vi "LabelNodeConfig.vi"(4 "State In":T1={"Name"="...", "Hash"=0, "Type"=enum."I32"}) -> (0 "Canceled?":bool, 1 "State Out":T1={"Name"="...", "Hash"=0, "Type"=enum."I32"})   [LabVIEW 2012]
uses:
  ScriptingSupport/PictureRing.ctl
  State.ctl
  Core/Master Types.ctl
  CRef.lvlib
  CRef Label Node.xnode
panel:
  out "VisibleLabel":string="0" caption="Updated Label:"
  in  "Type":T3=1 items=["Boolean"=1, "U32"=6, "I32"=7, "Single"=10]
  out "VisibleChecksum":string="0" caption="Checksum:"
  in  "Reference Label":string="{NULL}"
  in  "Cancel Button":bool
  in  "OK Button":bool
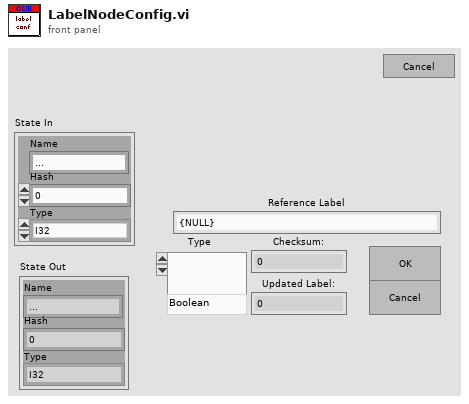
[diagram p1: front panel]
types:
  T1 = typedef "CRefScripting.lvlib/CRef Label Node.xnode/State.ctl" = cluster{"Name":string, "Hash":u32, "Type":T2}
  T2 = typedef "CRef.lvlib/Master Types.ctl" = enum8{"Null", "Boolean", "U8", "I8", "U16", "I16", "U32", "I32", "U64", "I64", "Single", "Double", "Extended", "CSG", "CDB", "CXT", "Boolean(Def)", "U8(Def)", "I8(Def)", "U16(Def)", "I16(Def)", "U32(Def)", "I32(Def)", "Reserved Def", "Reserved Def1", "Single(Def)", "Double(Def)", "Reserved Def2", "Reserved Def3", "Reserved Def4", "Reserved Def5", "Unsigned(Def)", "Signed(Def)", "Real(Def)", "Reserved Def6", "Numeric(Def)", "String"}
  T3 = typedef "CRef.lvlib/PictureRing.ctl" = u16
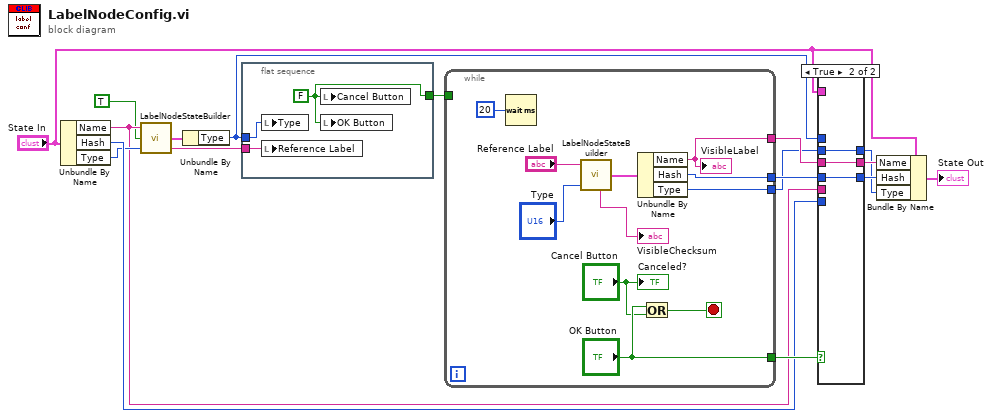
[diagram p0: block diagram]
diagram:
  n1 = Unbundle By Name("State In") -> ("Name"=w5:string, "Hash"=w7:u32, "Type"=w6:T2)
  n2 = call "LabelNodeStateBuilder.vi"("Reference Label"=w5, "Existing Label?"=TRUE, "Type"=w6) -> ("State Out"=w2:T1, "Cleaned Label"=w3:string)  [unwired: 4 in, 1 out]
  n3 = Unbundle By Name(w2) -> ("Type"=w1:T2)
  n4 = flat-sequence {
    tunnel: [w18] -> w17
    tunnel: w3 -> [w20]
    tunnel: w1 -> [w19]
    frame #0 {
      w18 = FALSE ("Cancel Button")
      n5 = local write "Type"(w19) -> ()
      n6 = local write "Reference Label"(w20) -> ()
      n7 = local write "Cancel Button"(w18) -> ()
      n8 = local write "OK Button"(w18) -> ()
    }
  }
  n9 = while {
    tunnel: w17 -> [_]
    tunnel: [w25] -> w15
    tunnel: ["OK Button"] -> w16
    tunnel: [w24] -> w14
    tunnel: [w26] -> w13
    stop <- w31 stop-if-true
    n10 = Wait (ms)(milliseconds to wait=u32 20) -> ()  [unwired: 1 out]
    n11 = call "LabelNodeStateBuilder.vi"("Reference Label"="Reference Label", "Type"="Type") -> ("State Out"=w27:T1, "VisibleChecksum"=→"VisibleChecksum":string)  [unwired: 5 in, 1 out]
    n12 = Unbundle By Name(w27) -> ("Name"=w24:string, "Hash"=w25:u32, "Type"=w26:T2)
    "VisibleLabel" <- w24
    n13 = Or(x="OK Button", y="Cancel Button") -> (x .or. y?=w31:bool)
    "Canceled?" <- "Cancel Button"
  }
  n14 = case shown="True" w16 {
    tunnel: w15 -> [_ w36]
    tunnel: w14 -> [_ w37]
    tunnel: w13 -> [_ w35]
    tunnel: [w34 w37] -> w12
    tunnel: [w33 w36] -> w11
    tunnel: [w32 w35] -> w10
    tunnel: "State In" -> [_ _]
    tunnel: w5 -> [w34 _]
    tunnel: w7 -> [w33 _]
    tunnel: w1 -> [w32 _]
    frame False {
    }
    frame True {
    }
  }
  n15 = Bundle By Name(cluster="State In", "Name"=w12, "Hash"=w11, "Type"=w10) -> (→"State Out":T1)
